vi "unwrap2D.vi"(9 "Array":dbl[][](array[numeric]), 10 "Numeric 2":i32, 11 "Numeric":i32) -> (3 "A + B":T1)   [LabVIEW 2015]
uses:
  <vilib>/Analysis/Matrix/Datatypes/RealMatrix.ctl
  <vilib>/Analysis/baseanly.llb/Real A x B.vi
  <vilib>/Analysis/Matrix/Numeric/Subtract/Subtract - RM,RM.vi
  <vilib>/Analysis/Matrix/Numeric/Add/Add - RM,RM.vi
  <vilib>/Analysis/Matrix/NI_Matrix.lvlib
  <vilib>/Analysis/NI_AALBase.lvlib
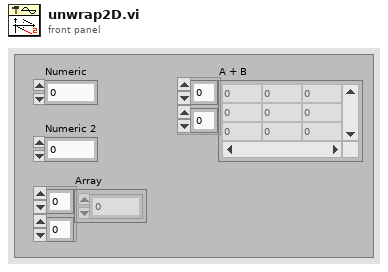
[diagram p1: front panel]
types:
  T1 = typedef "NI_Matrix.lvlib/RealMatrix.ctl" = dbl[][]
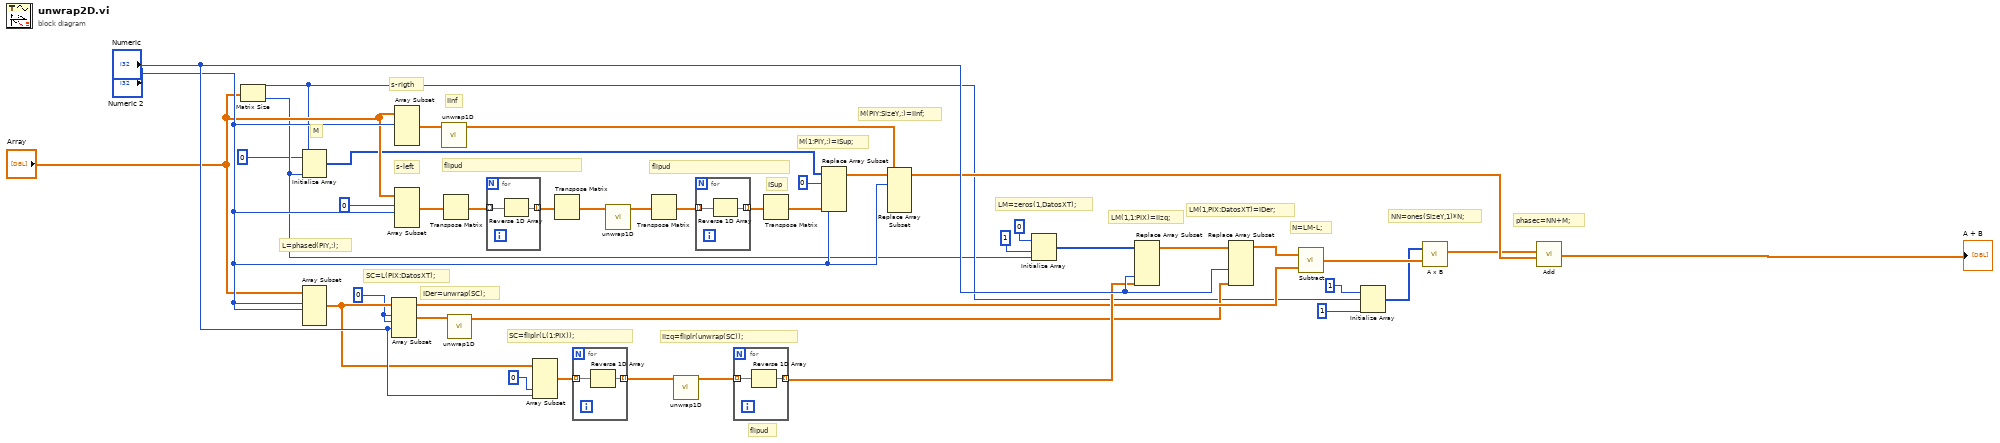
[diagram p0: block diagram]
diagram:
  w7 = 0
  # "N=LM-L;"
  # "LM(1,PIX:DatosXT)=IDer;"
  # "flipud"
  # "phasec=NN+M;"
  # "NN=ones(SizeY,1)*N;"
  # "IDer=unwrap(SC);"
  # "LM(1,1:PIX)=IIzq;"
  # "LM=zeros(1,DatosXT);"
  # "IIzq=fliplr(unwrap(SC));"
  # "flipud"
  # "SC=fliplr(L(1:PIX));"
  # "SC=L(PIX:DatosXT);"
  # "L=phased(PIY,:);"
  # "M(PIY:SizeY,:)=IInf;"
  # "M(1:PIY,:)=ISup;"
  # "M"
  # "ISup"
  # "flipud"
  # "s-left"
  # "s-rigth"
  # "IInf"
  n1 = Matrix Size(0:"Array") -> (1:w14:i32, 2:w10:i32)
  n2 = Initialize Array(0, w14, w10) -> (w4:i32[][])
  n3 = Array Subset(array="Array", index (row)="Numeric 2", length (row)="Numeric 2") -> (w29:dbl[][])  [unwired: 2 in]
  n4 = Array Subset(array=w29, index (row)=w7, length (row)=w7, index (col)="Numeric") -> (w27:dbl[][])  [unwired: 1 in]
  n5 = Array Subset(array="Array", index (row)="Numeric 2") -> (w1:dbl[][])  [unwired: 3 in]
  n6 = Array Subset(array="Array", index (row)=0, length (row)="Numeric 2") -> (w19:dbl[][])  [unwired: 2 in]
  n7 = call "unwrap1D.vi"("Array in"=w1) -> ("Array out"=w16:dbl[][])  [unwired: 10 in]
  n8 = Transpose Matrix(1:w19) -> (0:w20:dbl[][])
  n9 = call "unwrap1D.vi"("Array in"=w27) -> ("Array out"=w28:dbl[][])  [unwired: 10 in]
  n10 = for {
    tunnel: [w43] -> w17 mode=indexing
    tunnel: w20 -> [w42] mode=indexing
    n11 = Reverse 1D Array(array=w42) -> (reversed array=w43:dbl[])
  }
  n12 = Array Subset(array=w29, index (col)=0, length (col)="Numeric") -> (w30:dbl[][])  [unwired: 2 in]
  n13 = Transpose Matrix(1:w17) -> (0:w18:dbl[][])
  n14 = for {
    tunnel: w30 -> [w45] mode=indexing
    tunnel: [w44] -> w32 mode=indexing
    n15 = Reverse 1D Array(array=w45) -> (reversed array=w44:dbl[])
  }
  n16 = call "unwrap1D.vi"("Array in"=w18) -> ("Array out"=w21:dbl[][])  [unwired: 10 in]
  n17 = Transpose Matrix(1:w21) -> (0:w22:dbl[][])
  n18 = call "unwrap1D.vi"("Array in"=w32) -> ("Array out"=w25:dbl[][])  [unwired: 10 in]
  n19 = for {
    tunnel: w22 -> [w47] mode=indexing
    tunnel: [w46] -> w23 mode=indexing
    n20 = Reverse 1D Array(array=w47) -> (reversed array=w46:dbl[])
  }
  n21 = for {
    tunnel: w25 -> [w49] mode=indexing
    tunnel: [w48] -> w33 mode=indexing
    n22 = Reverse 1D Array(array=w49) -> (reversed array=w48:dbl[])
  }
  n23 = Transpose Matrix(1:w23) -> (0:w24:dbl[][])
  n24 = Replace Array Subset(array=w4, new element=w24, index (dim 0)=0, index (dim 1)="Numeric 2") -> (w6:T1)  [unwired: 2 in]
  n25 = Replace Array Subset(array=w6, new element=w16, index (dim 0)="Numeric 2") -> (w38:T1)  [unwired: 3 in]
  n26 = Initialize Array(0, 1, w10) -> (w11:i32[][])
  n27 = Replace Array Subset(array=w11, new element=w33, index (dim 3)="Numeric") -> (w26:T1)  [unwired: 3 in]
  n28 = Replace Array Subset(array=w26, new element=w28, index (dim 2)="Numeric") -> (w12:T1)  [unwired: 3 in]
  n29 = call-poly <vilib>:"Subtract.vi"("Real Matrix B"=w29, "Real Matrix A"=w12) -> ("A - B"=w36:T1)
  n30 = Initialize Array(1, w14, 1) -> (w35:i32[][])
  n31 = call-poly <vilib>:"A x B.vi"("B"=w36, "A"=w35) -> ("A x B"=w34:T1)  [unwired: 1 out]
  n32 = call-poly <vilib>:"Add.vi"("Real Matrix B"=w38, "Real Matrix A"=w34) -> ("A + B"=→"A + B":T1)
